vi "Shooter Angle.vi"(11 "AIDeviceRef":T1) -> (1 "Voltage":dbl, 2 "Shoter Angle":dbl)   [LabVIEW 2011]
uses:
  <vilib>/Rock Robotics/WPI/AnalogChannel/WPI_AnalogChannelDevRef.ctl
  <vilib>/Rock Robotics/SystemInterfaces/Typedef/FPGA_TypedefAnalogModule.ctl
  <vilib>/Rock Robotics/SystemInterfaces/AI/FPGA_AIChannel.ctl
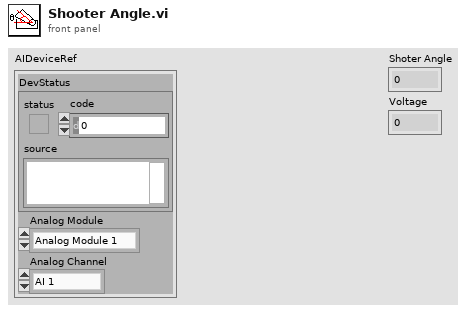
[diagram p1: front panel]
types:
  T1 = typedef "WPI_AnalogChannelDevRef.ctl" = cluster{"DevStatus":errorcluster, "Analog Module":T2, "Analog Channel":T3}
  T2 = typedef "FPGA_TypedefAnalogModule.ctl" = enum16{"Analog Module 1", "Analog Module 2"}
  T3 = typedef "FPGA_AIChannel.ctl" = enum8{"AI 1", "AI 2", "AI 3", "AI 4", "AI 5", "AI 6", "AI 7", "AI 8", "Invalid"}
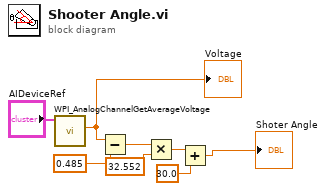
[diagram p0: block diagram]
diagram:
  n1 = call <vilib>:"WPI_AnalogChannelGetAverageVoltage.vi"("AIDeviceRef"="AIDeviceRef") -> ("Voltage"=w8:dbl)  [unwired: 8 in, 2 out]
  "Voltage" <- w8
  n2 = Subtract(x=w8, y=0.485) -> (x-y=w7:dbl)
  n3 = Multiply(x=w7, y=32.552) -> (x*y=w3:dbl)
  n4 = Add(x=w3, y=30.0) -> (x+y=→"Shoter Angle":dbl)
